vi "Consumer.vi"(8 "error in (no error)":errorcluster, 9 "Data":variant, 10 "Case ID":string, 11 "uService Template in":refnum<class "Run Config Manager.lvclass">) -> (0 "error out":errorcluster, 3 "uService Template out":refnum<class "Run Config Manager.lvclass">)   [LabVIEW 2026, in "TALOS.lvlib" / "Run Config Manager.lvlib" / "Run Config Manager.lvclass"]
uses:
  Run Config Manager.lvclass
  C:/LabVIEW Code/TALOS/talos/Father of all uServices/Father of all uServices/Father of all uServices.lvclass
  Run Config Manager Consumer Case Selector.ctl
  Ancestor/Ancestor/Ancestor.lvclass/Ancestor.ctl
  Support VIs/Generate Error.vi
  FGV/Error Memory/Get Error Description.vi
  Support VIs/Get PC name.vi
  Ancestor/Ancestor/Read ID.vi
  Support VIs/Get Class Name.vi
  <vilib>/Utility/error.llb/Clear Errors.vi
  FGV/Error Memory/Error Memory Core.vi
  <vilib>/AdvancedString/Delimited String to 1D String Array.vi
  <vilib>/AdvancedString/Delimited String to 1D String Array (string).vi
  FGV/Error Memory/Error Crt Lvl checker.vi
  FGV/Error Memory/Error Memory Core.vi/40c8088d-b597-4017-91af-faa98e00292e.vi
  FGV/Error Memory/Error Memory Core.vi/d4a3ab98-063c-4e44-b43d-fbdcfe6c2be2.vi
  Support VIs/Global Constants.vi
  Support VIs/Global Memory.vi
  <vilib>/Utility/LVClass/Get LV Class Name.vi
  Support VIs/Is in Packed Library.vi
  Support VIs/TALOS Root path.vi
  Support VIs/Read CSV worksheet.vi
  <vilib>/Utility/error.llb/General Error Handler.vi
  Support VIs/Error Log.vi
  Ancestor/Ancestor/Ancestor.lvclass
  <vilib>/Comparison/Equal/Equal Functor/Equal Functor.lvclass
  Father of all uServices/Father of all uServices/Father of all uServices.lvclass
  TALOS.lvlib
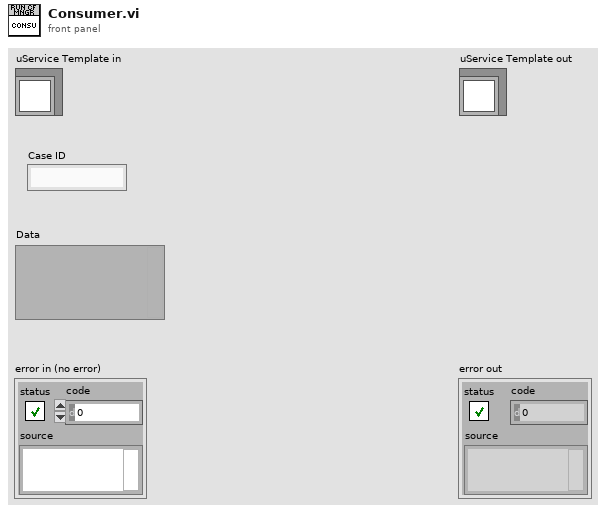
[diagram p1: front panel]
types:
  T1 = typedef "TALOS.lvlib/Run Config Manager.lvlib/Run Config Manager.lvclass/Run Config Manager Consumer Case Selector.ctl" = enum16{"Populate Run Config Ring"}
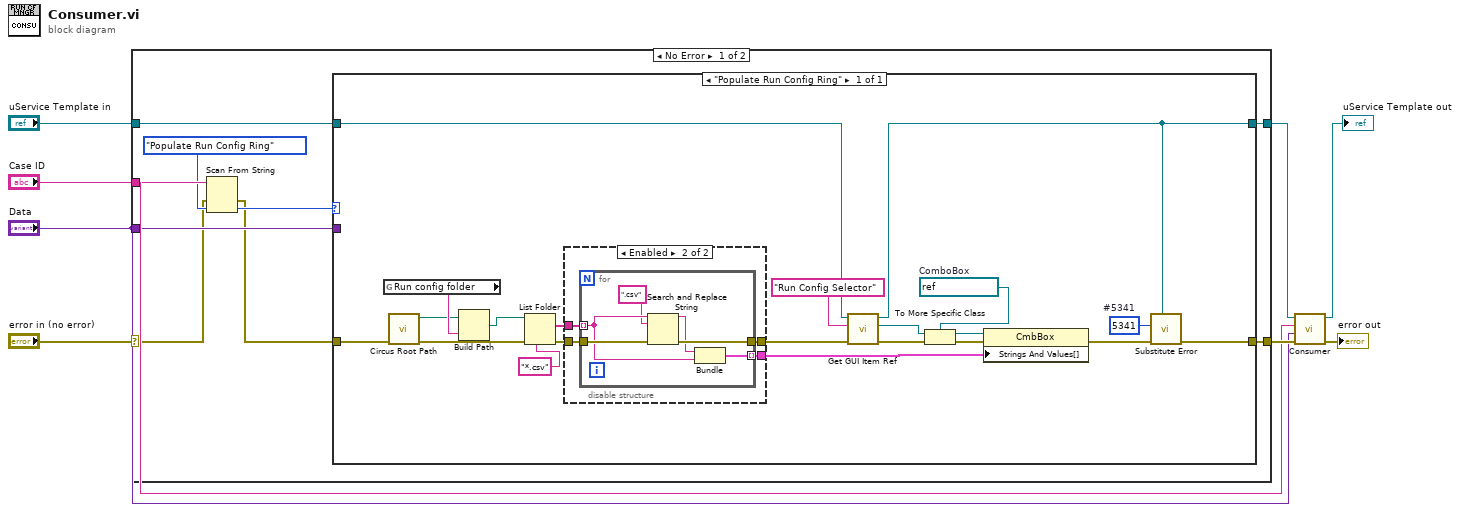
[diagram p0: block diagram]
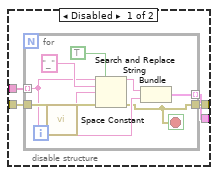
[diagram p2: hidden frame]
diagram:
  n1 = case shown="No Error" "error in (no error)" {
    selector: "error in (no error)" -> [w11 w61]
    tunnel: "uService Template in" -> [w16 w62]
    tunnel: [w9 w62] -> w4
    tunnel: [w15 w61] -> w3
    tunnel: "Case ID" -> [w14 _]
    tunnel: "Data" -> [w17 _]
    frame No Error {
      n2 = Scan From String(input string=w14, error in=w11, default 1=Run_Config_Manager_Consumer_Case_Selector."Populate Run Config Ring") -> (error out=w10:errorcluster, output 1=w12:T1)  [unwired: 2 in, 2 out]
      n3 = case shown="\"Populate Run Config Ring\"" w12 {
        tunnel: w17 -> [_]
        tunnel: w10 -> [w21]
        tunnel: w16 -> [w19]
        tunnel: [w20] -> w15
        tunnel: [w18] -> w9
        frame "Populate Run Config Ring" {
          w25 = 5341  # #5341
          w24 = refnum<vi> refnum  # ComboBox
          n4 = global read "Global Constants.vi" "Run config folder"() -> (w27:string)
          n5 = call "Circus Root Path.vi"("error in (no error)"=w21) -> ("error out"=w28:errorcluster, "Circus Root Path"=w26:path)  [unwired: 9 in]
          n6 = Build Path(base path=w26, name or relative path=w27) -> (appended path=w29:path)
          n7 = List Folder(path=w29, pattern="*.csv", error in=w28) -> (filenames=w35:string[], error out=w34:errorcluster)  [unwired: 1 in, 2 out]
          n8 = disable-structure shown="Enabled" {
            disable-tunnel: w34 -> [w42 w54]
            disable-tunnel: w35 -> [w41 w53]
            disable-tunnel: [w40 w52] -> w36
            disable-tunnel: [w39 w51] -> w37
            frame Disabled {
              n9 = for {
                tunnel: w42 -> [w50]
                tunnel: w41 -> [w45] mode=indexing
                tunnel: [w44] -> w39 mode=indexing
                tunnel: [w43] -> w40
                stop <- w43 stop-if-true
                n10 = call <vilib>:"Space Constant.vi"() -> ("String"=w47:string)
                n11 = Search and Replace String(replace all?=TRUE ("replace all? (F)"), input string=w45, search string="_", replace string=w47, error in=w50) -> (result string=w46:string, error out=w43:errorcluster)  [unwired: 3 in, 2 out]
                n12 = Bundle(w46, w45) -> (w44:cluster{string, string})  [unwired: 1 in]
              }
            }
            frame Enabled {
              n13 = for {
                tunnel: w54 -> [w59]
                tunnel: w53 -> [w56] mode=indexing
                tunnel: [w60] -> w51 mode=indexing
                tunnel: [w58] -> w52
                n14 = Search and Replace String(input string=w56, search string=".csv", error in=w59) -> (result string=w57:string, error out=w58:errorcluster)  [unwired: 5 in, 2 out]
                n15 = Bundle(w57, w56) -> (w60:cluster{string, string})  [unwired: 1 in]
              }
            }
          }
          n16 = call "Get GUI Item Ref.vi"("error in (no error)"=w36, "FP Item Name"="Run Config Selector", "uService Template in"=w19) -> ("error out"=w30:errorcluster, "Ctl Refnum"=w32:refnum<vi>, "uService Template out"=w18:refnum<class "Run Config Manager.lvclass">)  [unwired: 6 in]
          n17 = To More Specific Class(target class=w24, reference=w32, error in=w30) -> (specific class reference=w33:refnum<vi>, error out=w31:errorcluster)
          n18 = property class="CmbBox"(reference=w33, error in=w31, "Strings And Values[]"=w37) -> (error out=w38:errorcluster)  [unwired: 1 out]
          n19 = call "Substitute Error.vi"("LabVIEW Object"=w18, "error in (no error)"=w38, "Error Code"=w25) -> ("error out"=w20:errorcluster)  [unwired: 8 in]
        }
      }
    }
    frame Error {
    }
  }
  n20 = call-parent "Consumer.vi"("error in (no error)"=w3, "Data"="Data", "Case ID"="Case ID", "uService Template in"=w4) -> ("error out"=→"error out":errorcluster, "uService Template out"=→"uService Template out":refnum<class "Run Config Manager.lvclass">)  [unwired: 6 in]
